vi "Single Freq Gen.vi"(7 "Stop Single Frquency":bool, 10 "Amplitude":T1, 11 "Frequency (MHz)":T2) -> (1 "Hex String 2":string, 3 "Hex String 1":string)   [LabVIEW 2017]
uses:
  TypeDef/Frequency.ctl
  TypeDef/Amplitude.ctl
  Globals/FPGA Globals.vi
panel:
  out "Hex Length 2":i32
  out "Hex Length 1":i32
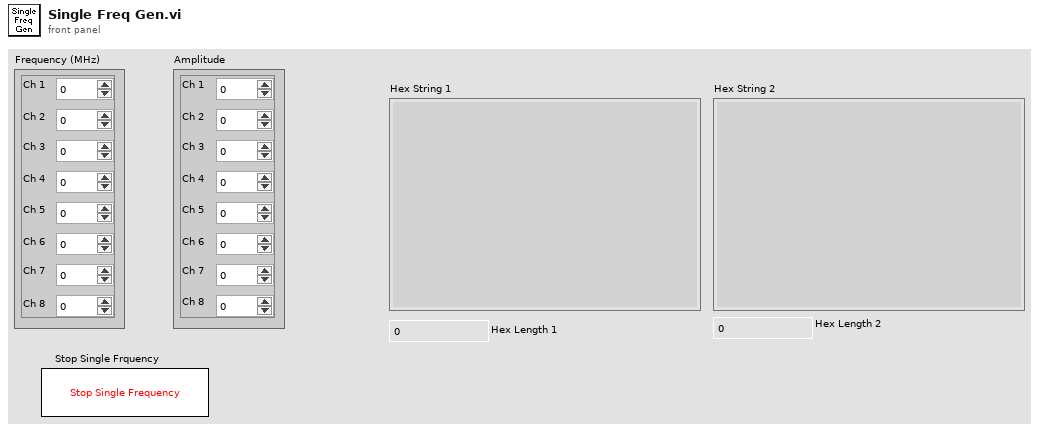
[diagram p1: front panel]
types:
  T1 = typedef "Amplitude.ctl" = cluster{"Ch 1":u16, "Ch 2":u16, "Ch 3":u16, "Ch 4":u16, "Ch 5":u16, "Ch 6":u16, "Ch 7":u16, "Ch 8":u16}
  T2 = typedef "Frequency.ctl" = cluster{"Ch 1":u16, "Ch 2":u16, "Ch 3":u16, "Ch 4":u16, "Ch 5":u16, "Ch 6":u16, "Ch 7":u16, "Ch 8":u16}
  T3 = typedef "FPGA Settings.ctl" = cluster{"System Clock(MHz)":dbl, "FPGA MAC 1":string, "Port Number 1":i32, "Port Number 2":i32, "FPGA MAC 2":string}
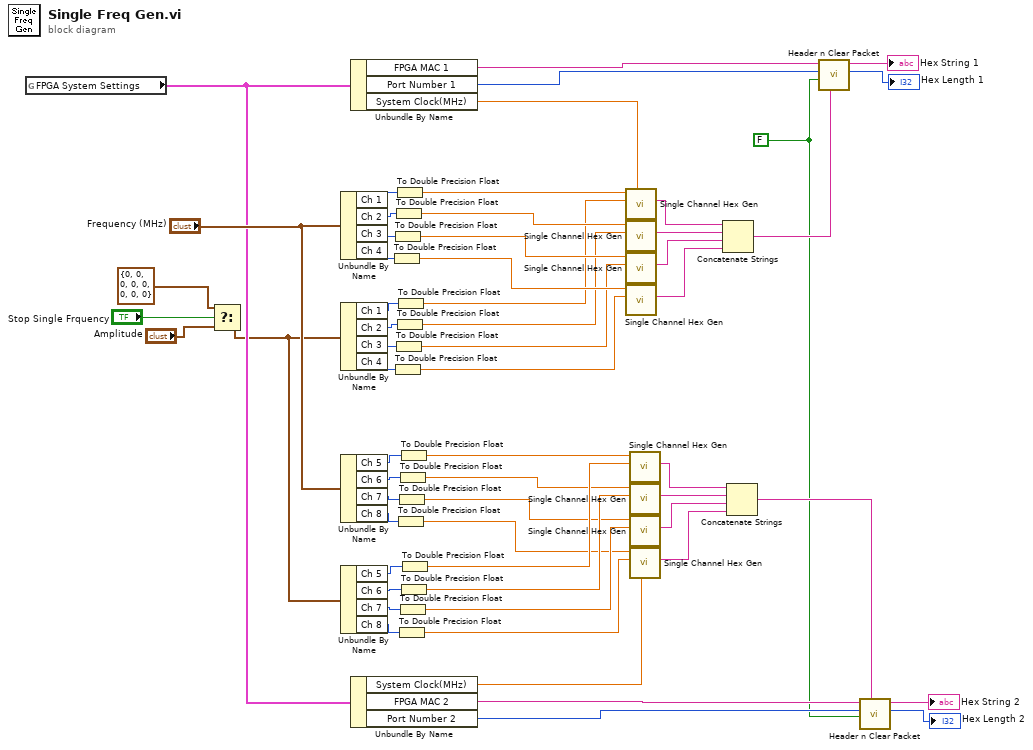
[diagram p0: block diagram]
diagram:
  w5 = FALSE ("Stop Single Frquency")
  n1 = global read "FPGA Globals.vi" "FPGA System Settings"() -> (w6:T3)
  n2 = Select(t=T1 {"Ch 1"=0, "Ch 2"=0, "Ch 3"=0, "Ch 4"=0, "Ch 5"=0, "Ch 6"=0, "Ch 7"=0, "Ch 8"=0}, s="Stop Single Frquency", f="Amplitude") -> (s? t:f=w1:T1)
  n3 = Unbundle By Name("Frequency (MHz)") -> ("Ch 1"=w55:u16, "Ch 2"=w53:u16, "Ch 3"=w51:u16, "Ch 4"=w49:u16)
  n4 = Unbundle By Name(w1) -> ("Ch 1"=w44:u16, "Ch 2"=w45:u16, "Ch 3"=w46:u16, "Ch 4"=w47:u16)
  n5 = Unbundle By Name("Frequency (MHz)") -> ("Ch 5"=w24:u16, "Ch 6"=w26:u16, "Ch 7"=w28:u16, "Ch 8"=w30:u16)
  n6 = Unbundle By Name(w1) -> ("Ch 5"=w35:u16, "Ch 6"=w34:u16, "Ch 7"=w33:u16, "Ch 8"=w32:u16)
  n7 = Unbundle By Name(w6) -> ("FPGA MAC 1"=w12:string, "Port Number 1"=w11:i32, "System Clock(MHz)"=w7:dbl)
  n8 = Unbundle By Name(w6) -> ("System Clock(MHz)"=w8:dbl, "FPGA MAC 2"=w10:string, "Port Number 2"=w9:i32)
  n9 = To Double Precision Float(number=w49) -> (double precision float=w48:dbl)
  n10 = To Double Precision Float(number=w51) -> (double precision float=w50:dbl)
  n11 = To Double Precision Float(number=w47) -> (double precision float=w40:dbl)
  n12 = To Double Precision Float(number=w53) -> (double precision float=w52:dbl)
  n13 = To Double Precision Float(number=w46) -> (double precision float=w41:dbl)
  n14 = To Double Precision Float(number=w55) -> (double precision float=w54:dbl)
  n15 = To Double Precision Float(number=w45) -> (double precision float=w42:dbl)
  n16 = To Double Precision Float(number=w44) -> (double precision float=w43:dbl)
  n17 = To Double Precision Float(number=w30) -> (double precision float=w31:dbl)
  n18 = To Double Precision Float(number=w28) -> (double precision float=w29:dbl)
  n19 = To Double Precision Float(number=w32) -> (double precision float=w39:dbl)
  n20 = To Double Precision Float(number=w26) -> (double precision float=w27:dbl)
  n21 = To Double Precision Float(number=w33) -> (double precision float=w38:dbl)
  n22 = To Double Precision Float(number=w24) -> (double precision float=w25:dbl)
  n23 = To Double Precision Float(number=w34) -> (double precision float=w37:dbl)
  n24 = To Double Precision Float(number=w35) -> (double precision float=w36:dbl)
  n25 = call "Single Channel Hex Gen.vi"("System Clock(MHz)"=w7, "Amplitude"=w43, "Frequency"=w54) -> ("Single Freq Hex String"=w59:string)  [unwired: 8 in]
  n26 = call "Single Channel Hex Gen.vi"("System Clock(MHz)"=w7, "Amplitude"=w42, "Frequency"=w52) -> ("Single Freq Hex String"=w58:string)  [unwired: 8 in]
  n27 = call "Single Channel Hex Gen.vi"("System Clock(MHz)"=w7, "Amplitude"=w41, "Frequency"=w50) -> ("Single Freq Hex String"=w57:string)  [unwired: 8 in]
  n28 = call "Single Channel Hex Gen.vi"("System Clock(MHz)"=w7, "Amplitude"=w40, "Frequency"=w48) -> ("Single Freq Hex String"=w56:string)  [unwired: 8 in]
  n29 = call "Single Channel Hex Gen.vi"("System Clock(MHz)"=w8, "Amplitude"=w36, "Frequency"=w25) -> ("Single Freq Hex String"=w20:string)  [unwired: 8 in]
  n30 = call "Single Channel Hex Gen.vi"("System Clock(MHz)"=w8, "Amplitude"=w37, "Frequency"=w27) -> ("Single Freq Hex String"=w21:string)  [unwired: 8 in]
  n31 = call "Single Channel Hex Gen.vi"("System Clock(MHz)"=w8, "Amplitude"=w38, "Frequency"=w29) -> ("Single Freq Hex String"=w22:string)  [unwired: 8 in]
  n32 = call "Single Channel Hex Gen.vi"("System Clock(MHz)"=w8, "Amplitude"=w39, "Frequency"=w31) -> ("Single Freq Hex String"=w23:string)  [unwired: 8 in]
  n33 = Concatenate Strings(w59, w58, w57, w56) -> (w16:string)
  n34 = Concatenate Strings(w20, w21, w22, w23) -> (w13:string)
  n35 = call "Header n Clear Packet.vi"("Hex String in"=w16, "Stop Single Frquency"=w5, "Port Number"=w11, "FPGA MAC"=w12) -> ("Hex Length"=→"Hex Length 1":i32, "Hex String out"=→"Hex String 1":string)  [unwired: 6 in]
  n36 = call "Header n Clear Packet.vi"("Hex String in"=w13, "Stop Single Frquency"=w5, "Port Number"=w9, "FPGA MAC"=w10) -> ("Hex Length"=→"Hex Length 2":i32, "Hex String out"=→"Hex String 2":string)  [unwired: 6 in]
